vi "crab drive.vi"() -> ()   [LabVIEW 2009]
uses:
  crabe drive.ctl
panel:
  out "wheels":cluster{"speed":dbl, "direction":dbl}[](array[cluster]) {"direction" scale=0.0..6.3; "speed" scale=-1.0..1.0}
  in  "user control":T1 {"turn" scale=-1.0..1.0; "skew (direction)" scale=0.0..6.28318470517958 scale format="%.1g"; "speed" scale=-1.0..1.0}
  # "ignore \"skew rate\" for now"
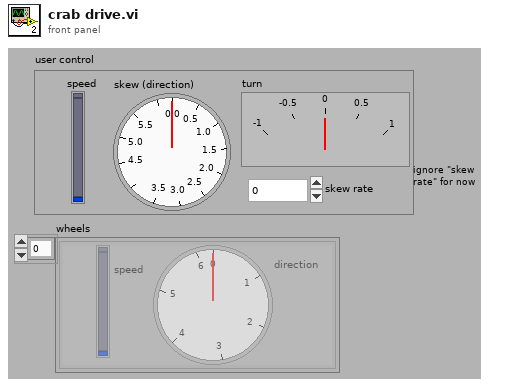
[diagram p1: front panel]
types:
  T1 = typedef "crabe drive.ctl" = cluster{"speed":dbl, "skew (direction)":dbl, "turn":dbl, "skew rate":dbl}
  T2 = enum8{"none", "descel only", "accel only", "both"}
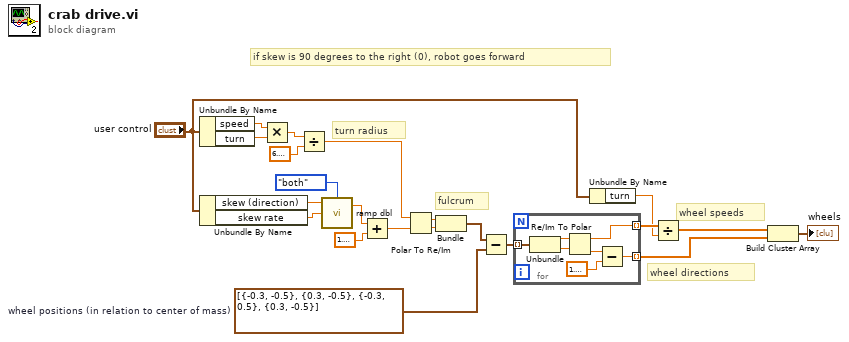
[diagram p0: block diagram]
diagram:
  w15 = cluster{dbl, dbl}[] [{-0.3, -0.5}, {0.3, -0.5}, {-0.3, 0.5}, {0.3, -0.5}]  # wheel positions (in relation to center of mass)
  # "wheel speeds"
  # "wheel directions"
  # "if skew is 90 degrees to the right (0), robot goes forward"
  # "fulcrum"
  # "turn radius"
  n1 = Unbundle By Name("user control") -> ("speed"=w22:dbl, "turn"=w21:dbl)
  n2 = Unbundle By Name("user control") -> ("skew (direction)"=w11:dbl, "skew rate"=w10:dbl)
  n3 = Multiply(x=w22, y=w21) -> (x*y=w20:dbl)
  n4 = Divide(x=w20, y=6.283185307179586) -> (x/y=w18:dbl)
  n5 = call "ramp dbl.vi"("ramp mode"=T2."both", "max change/s"=w10, "setpoint"=w11) -> ("output"=w3:dbl)  [unwired: 1 in, 1 out]
  n6 = Add(x=w3, y=1.5707963267948966) -> (x+y=w1:dbl)
  n7 = Polar To Re/Im(2:w1, 3:w18) -> (0:w16:dbl, 1:w17:dbl)
  n8 = Bundle(w17, w16) -> (w14:cluster{dbl, dbl})  [unwired: 1 in]
  n9 = Subtract(x=w14, y=w15) -> (x-y=w13:cluster{dbl, dbl}[])
  n10 = for {
    tunnel: w13 -> [w29] mode=indexing
    tunnel: [w26] -> w8 mode=indexing
    tunnel: [w23] -> w6 mode=indexing
    n11 = Unbundle(w29) -> (w27:dbl, w28:dbl)
    n12 = Re/Im To Polar(2:w28, 3:w27) -> (0:w25:dbl, 1:w26:dbl)
    n13 = Subtract(x=w25, y=1.5707963267948966) -> (x-y=w23:dbl)
  }
  n14 = Unbundle By Name("user control") -> ("turn"=w7:dbl)
  n15 = Divide(x=w8, y=w7) -> (x/y=w5:dbl[])
  n16 = Build Cluster Array(w5, w6) -> (→"wheels":cluster{dbl, dbl}[])
